vi "Clean Up Actor.vi"(8 "error in (no error)":errorcluster, 11 "Terminal Menus in":refnum<class "Terminal Menus.lvclass">) -> (0 "error out":errorcluster, 3 "Terminal Menus out":refnum<class "Terminal Menus.lvclass">)   [LabVIEW 2016, in "CLD Exam - ATM.lvlib" / "Terminal Menus.lvclass"]
uses:
  Terminal Menus.lvclass
  D:/Repos/Stream/software/Mediator/Classes/Mediated Actor/Mediated Actor.lvclass
  Mediator/Classes/Message Broker Interface/Message Broker Interface.lvclass
  Mediator/Classes/Mediated Synchronous Actor/Mediated Synchronous Actor.lvclass
  Mediator/Classes/Mediated Actor/Mediated Actor.lvclass
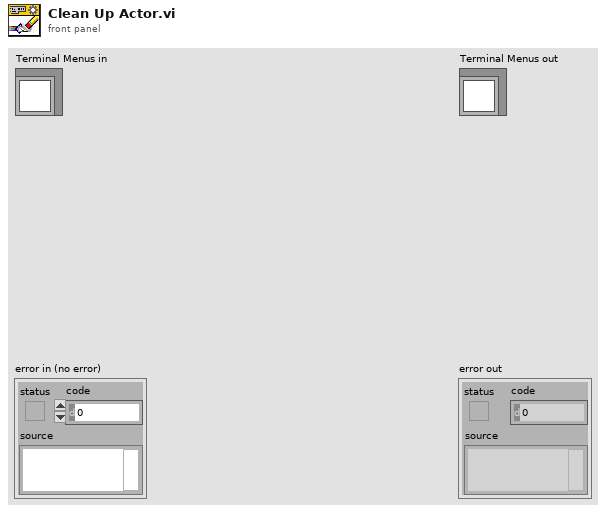
[diagram p1: front panel]
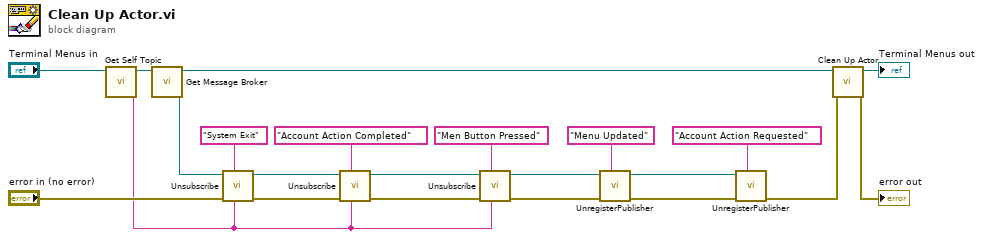
[diagram p0: block diagram]
diagram:
  n1 = call "Get Self Topic.vi"("Mediated Actor in"="Terminal Menus in") -> ("Topic.Self"=w8:string, "Mediated Actor out"=w20:refnum<class "Terminal Menus.lvclass">)  [unwired: 9 in]
  n2 = call "Get Message Broker.vi"("Mediated Actor in"=w20) -> ("Message Broker"=w11:refnum<class "Message Broker Interface.lvclass">, "Mediated Actor out"=w18:refnum<class "Terminal Menus.lvclass">)  [unwired: 9 in]
  n3 = call-dynamic "Unsubscribe.vi"("Subscriber Name"=w8, "Topic Name"="System Exit", "error in (no error)"="error in (no error)", "Message Broker Interface in"=w11) -> ("error out"=w14:errorcluster, "Message Broker Interface out"=w13:refnum<class "Message Broker Interface.lvclass">)  [unwired: 6 in]
  n4 = call-dynamic "Unsubscribe.vi"("Subscriber Name"=w8, "Topic Name"="Account Action Completed", "error in (no error)"=w14, "Message Broker Interface in"=w13) -> ("error out"=w7:errorcluster, "Message Broker Interface out"=w9:refnum<class "Message Broker Interface.lvclass">)  [unwired: 6 in]
  n5 = call-dynamic "Unsubscribe.vi"("Subscriber Name"=w8, "Topic Name"="Men Button Pressed", "error in (no error)"=w7, "Message Broker Interface in"=w9) -> ("error out"=w5:errorcluster, "Message Broker Interface out"=w6:refnum<class "Message Broker Interface.lvclass">)  [unwired: 6 in]
  n6 = call-dynamic "UnregisterPublisher.vi"("Topic Name"="Menu Updated", "error in (no error)"=w5, "Message Broker Interface in"=w6) -> ("error out"=w3:errorcluster, "Message Broker Interface out"=w1:refnum<class "Message Broker Interface.lvclass">)  [unwired: 7 in]
  n7 = call-dynamic "UnregisterPublisher.vi"("Topic Name"="Account Action Requested", "error in (no error)"=w3, "Message Broker Interface in"=w1) -> ("error out"=w2:errorcluster)  [unwired: 7 in, 1 out]
  n8 = call-parent "Clean Up Actor.vi"("error in (no error)"=w2, "Mediated Actor in"=w18) -> ("error out"=→"error out":errorcluster, "Mediated Actor out"=→"Terminal Menus out":refnum<class "Terminal Menus.lvclass">)  [unwired: 8 in]
